vi "411x_Create I Chans.vi"(5 "Device Ref in":T1 format="%.0x", 7 "# of I Channels to Add?":i16, 8 "error in":errorcluster, 9 "sense":T2=1008 caption="sense (out)" items=["Local"=1008, "Remote"=1009], 10 "Voltage Limit":dbl, 11 "Init Value":dbl) -> (0 "error out":errorcluster)   [LabVIEW 2023, in "NI PXIe-411x PS Custom Device.lvlib"]
uses:
  NI PXIe-411x PS Custom Device.lvlib
  <instrlib>/niDCPower/nidcpower.llb/niDCPower Sense.ctl
  <vilib>/NI VeriStand/Custom Device API/Custom Device Item Ref.ctl
  <vilib>/NI VeriStand/Custom Device API/Custom Device Channel.ctl
  <vilib>/NI VeriStand/Custom Device API/Custom Device Channel Type.ctl
  411x_Global.vi
  <vilib>/NI VeriStand/Custom Device API/Get Item Property (U16).vi
  <vilib>/NI VeriStand/Custom Device API/Get Item Property (Boolean).vi
  <vilib>/NI VeriStand/Custom Device API/Set Item Property (U16).vi
  <vilib>/NI VeriStand/Custom Device API/Custom Device API.lvlib
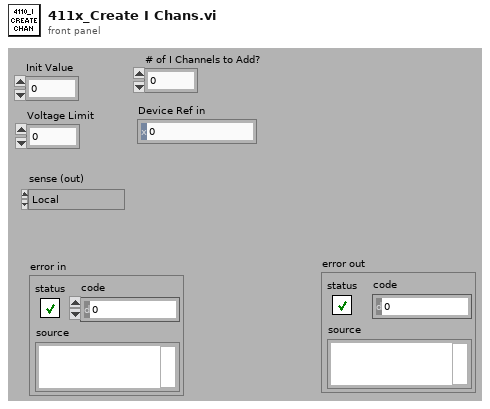
[diagram p1: front panel]
types:
  T1 = typedef "Custom Device API.lvlib/Custom Device Item Ref.ctl" = u64
  T2 = typedef "niDCPower Sense.ctl" = i32
  T3 = typedef "Custom Device API.lvlib/Custom Device Channel.ctl" = cluster{"Type":T4, "Units":string, "Default Value":dbl, "Faultable":bool, "Scalable":bool}
  T4 = typedef "Custom Device API.lvlib/Custom Device Channel Type.ctl" = enum16{"Input", "Output"}
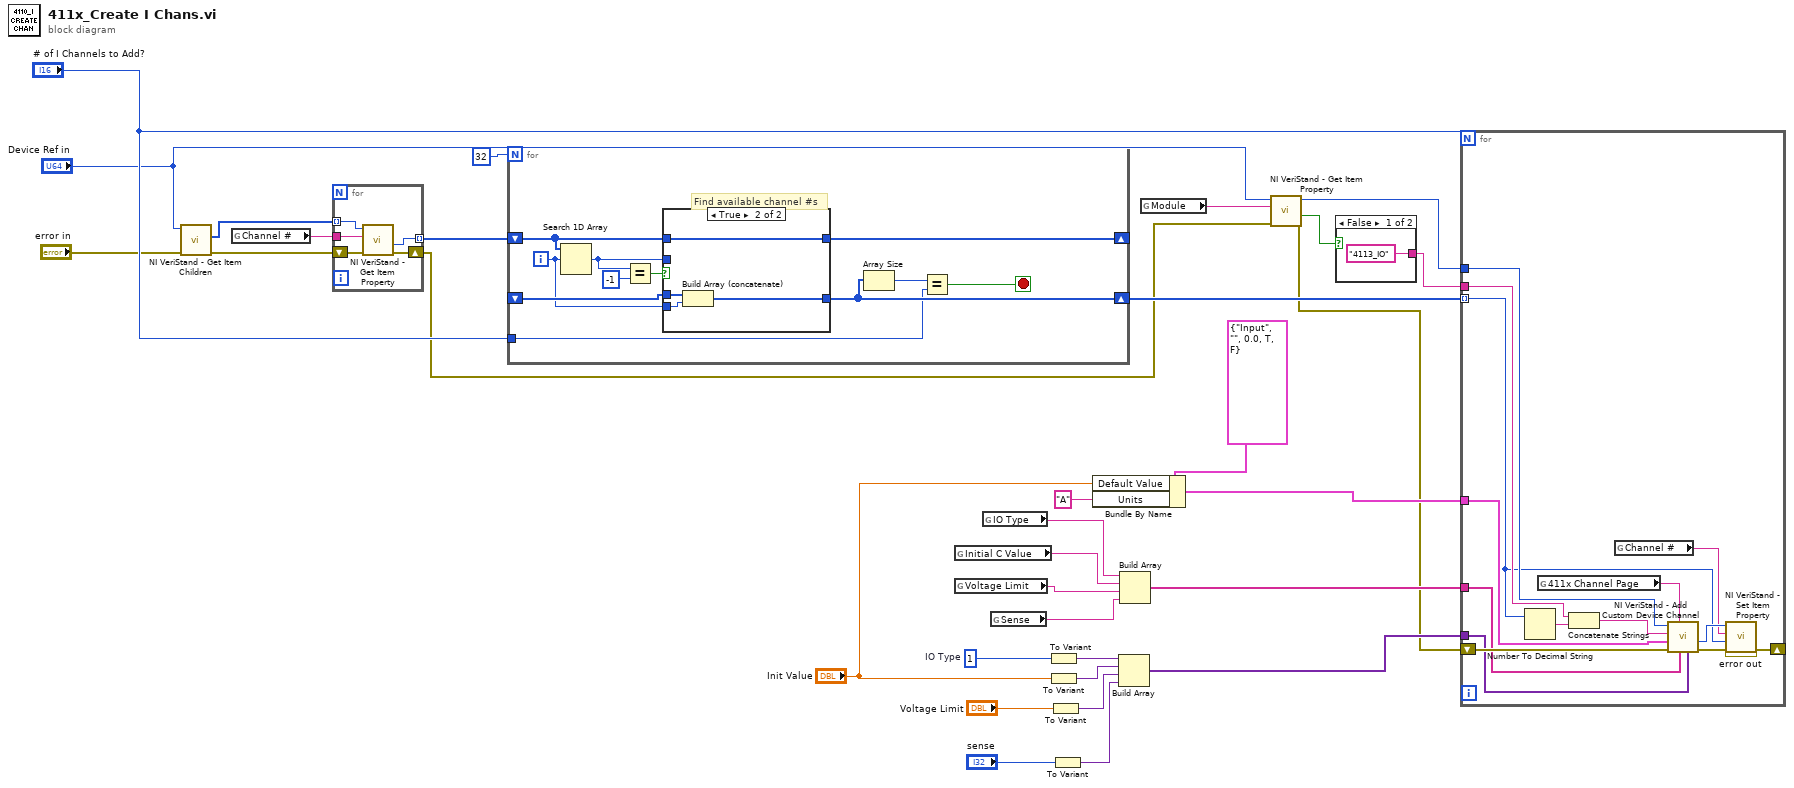
[diagram p0: block diagram]
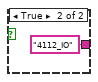
[diagram p2: hidden frame]
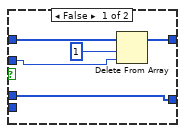
[diagram p3: hidden frame]
diagram:
  w11 = u16 1  # IO Type
  n1 = call <vilib>:"NI VeriStand - Get Item Children.vi"("error in (no error)"="error in", "Item Ref in"="Device Ref in") -> ("error out"=w23:errorcluster, "Child Refs"=w24:T1[])  [unwired: 6 in, 2 out]
  n2 = global read "411x_Global.vi" "Channel #"() -> (w16:string)
  n3 = for {
    tunnel: w24 -> [w38] mode=indexing
    shift-right: [w35] -> w4
    shift-left: w23 -> [w37]
    tunnel: w16 -> [w36]
    tunnel: [w34] -> w22 mode=indexing
    n4 = call-poly <vilib>:"NI VeriStand - Get Item Property.vi"("error in (no error)"=w37, "Property Name"=w36, "Item Ref in"=w38) -> ("error out"=w35:errorcluster, "Value"=w34:u16)  [unwired: 5 in, 2 out]
  }
  n5 = for {
    N: 32 -> [_]
    shift-right: [w42] -> w21
    shift-left: _ -> [w47]
    shift-right: [w43] -> _
    shift-left: w22 -> [w45]
    tunnel: "# of I Channels to Add?" -> [w40]
    i -> [w46]
    stop <- w39 stop-if-true
    # "Find available channel #s"
    n6 = Search 1D Array(1D array=w45, element=w46) -> (index of element=w44:i32)  [unwired: 1 in]
    n7 = Equal?(x=w44, y=-1) -> (x = y?=w48:bool)
    n8 = case shown="True" w48 {
      tunnel: w47 -> [w54 w58]
      tunnel: [w54 w57] -> w42
      tunnel: w46 -> [_ w56]
      tunnel: w45 -> [w53 w55]
      tunnel: w44 -> [w51 _]
      tunnel: [w50 w55] -> w43
      frame False {
        n9 = Delete From Array(array=w53, length=1, index=w51) -> (array with subset deleted=w50:u16[])  [unwired: 1 out]
      }
      frame True {
        n10 = Build Array (concatenate)(w58, w56) -> (w57:i32[])
      }
    }
    n11 = Array Size(array=w42) -> (size(s)=w41:i32)
    n12 = Equal?(x=w41, y=w40) -> (x = y?=w39:bool)
  }
  n13 = global read "411x_Global.vi" "Initial C Value"() -> (w14:string)
  n14 = global read "411x_Global.vi" "Voltage Limit"() -> (w13:string)
  n15 = global read "411x_Global.vi" "IO Type"() -> (w15:string)
  n16 = global read "411x_Global.vi" "Sense"() -> (w12:string)
  n17 = To Variant(anything=w11) -> (Variant=w28:variant)
  n18 = To Variant(anything="Init Value") -> (Variant=w29:variant)
  n19 = To Variant(anything="Voltage Limit") -> (Variant=w30:variant)
  n20 = To Variant(anything="sense") -> (Variant=w31:variant)
  n21 = Bundle By Name(cluster=T3 {"Type"=enum."Input", "Units"="", "Default Value"=0.0, "Faultable"=TRUE, "Scalable"=FALSE} ("Channel"), "Default Value"="Init Value", "Units"="A") -> (w19:T3)
  n22 = Build Array(w28, w29, w30, w31) -> (w32:variant[])
  n23 = Build Array(w15, w14, w13, w12) -> (w33:string[])
  n24 = global read "411x_Global.vi" "Module"() -> (w6:string)
  n25 = call-poly <vilib>:"NI VeriStand - Get Item Property.vi"("error in (no error)"=w4, "Property Name"=w6, "Item Ref in"="Device Ref in") -> ("error out"=w1:errorcluster, "Value"=w3:bool, "Item Ref out"=w2:T1)  [unwired: 5 in, 1 out]
  n26 = case shown="False" w3 {
    tunnel: ["4113_IO" "4112_IO"] -> w27
    frame False {
    }
    frame True {
    }
  }
  n27 = for {
    N: "# of I Channels to Add?" -> [_]
    shift-right: [w67] -> w26
    shift-left: w1 -> [w74]
    tunnel: w19 -> [w73]
    tunnel: w2 -> [w72]
    tunnel: w27 -> [w71]
    tunnel: w32 -> [w65]
    tunnel: w33 -> [w64]
    tunnel: w21 -> [w63] mode=indexing
    n28 = Number To Decimal String(number=w63) -> (decimal integer string=w70:string)  [unwired: 1 in]
    n29 = global read "411x_Global.vi" "411x Channel Page"() -> (w61:string)
    n30 = Concatenate Strings(w71, w70) -> (w69:string)
    n31 = global read "411x_Global.vi" "Channel #"() -> (w62:string)
    n32 = call <vilib>:"NI VeriStand - Add Custom Device Channel.vi"("Property Values"=w65, "Property names"=w64, "GUID (Default Channel)"=w61, "error in (no error)"=w74, "Channel"=w73, "Channel Name"=w69, "Parent Ref in"=w72) -> ("error out"=w68:errorcluster, "Channel Ref"=w66:T1)  [unwired: 1 in, 2 out]
    n33 = call-poly <vilib>:"NI VeriStand - Set Item Property.vi"("error in (no error)"=w68, "Value"=w63, "Property Name"=w62, "Item Ref in"=w66) -> ("error out"=w67:errorcluster)  [unwired: 5 in, 2 out]
  }
  "error out" <- w26
